vi "getDTFromXmlNative.vi"(8 "error in (no error)":errorcluster, 10 "eventXML":refnum<k20>, 11 "ScriptEvent in":refnum<class "ScriptEvent.lvclass">) -> (0 "error out":errorcluster, 2 "eventXML out":refnum<k20>, 3 "ScriptEvent out":refnum<class "ScriptEvent.lvclass">)   [LabVIEW 2009, in "Tools.lvlib" / "Scripting.lvlib" / "ScriptEvent.lvclass"]
uses:
  ScriptEvent.lvclass
  <vilib>/xml/Close Reference(Node).vi
  ScriptEvent.lvclass/ScriptEvent.ctl
  <vilib>/xml/NI_XML.lvlib
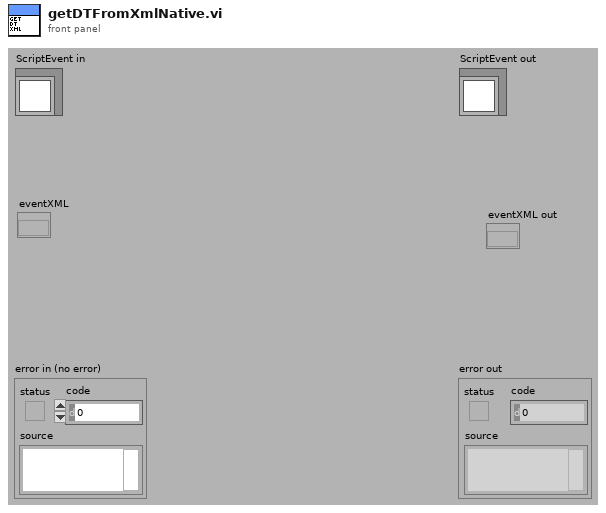
[diagram p1: front panel]
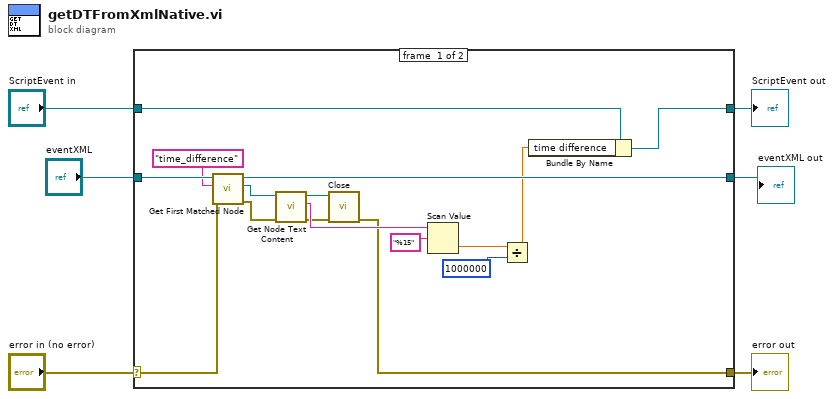
[diagram p0: block diagram]
diagram:
  n1 = case shown="No Error" "error in (no error)" {
    selector: "error in (no error)" -> [w7 w24]
    tunnel: [w8 w24] -> w5
    tunnel: [w9 w23] -> w3
    tunnel: "ScriptEvent in" -> [w10 w23]
    tunnel: "eventXML" -> [w22 _]
    tunnel: [w12 _] -> w1
    frame #0 {
      n2 = call <vilib>:"Get First Matched Node.vi"("error in (no error)"=w7, "XPath expression"="time_difference", "node in"=w22) -> ("error out"=w17:errorcluster, "node result"=w16:refnum<k20>, "node out"=w12:refnum<k20>)  [unwired: 6 in]
      n3 = call <vilib>:"Get Node Text Content.vi"("error in (no error)"=w17, "node in"=w16) -> ("error out"=w14:errorcluster, "node text"=w15:string, "node out"=w13:refnum<k20>)  [unwired: 7 in]
      n4 = call-poly <vilib>:"Close.vi"("error in (no error)"=w14, "node"=w13) -> ("error out"=w8:errorcluster)  [unwired: 7 in]
      n5 = Scan Value(string=w15, format string="%15") -> (value=w18:dbl)  [unwired: 1 in, 1 out]
      n6 = Divide(x=w18, y=1000000) -> (x/y=w11:dbl)
      n7 = Bundle By Name(cluster=w10, "time difference"=w11) -> (w9:refnum<class "ScriptEvent.lvclass">)
    }
    frame #1 {
    }
  }
  "error out" <- w5
  "ScriptEvent out" <- w3
  "eventXML out" <- w1
